vi "Wait Event Callback.vi"(4 "GUI.lvlib:Auto UI.lvlib:Auto UI.lvclass":refnum<class "Auto UI.lvclass">, 5 "Event data":cluster{"showWait":bool}, 6 "CtlRef":refnum<k7>, 7 "Event common data":cluster{"Source":i32, "Type":u32, "Time":u32}) -> ()   [LabVIEW 2023, in "GUI.lvlib" / "Auto UI.lvlib" / "Auto UI.lvclass"]
uses:
  Auto UI.lvclass
  Auto UI.lvclass/Auto UI.ctl
  <vilib>/Utility/cursorutil.llb/Set Cursor (Icon Pict).vi
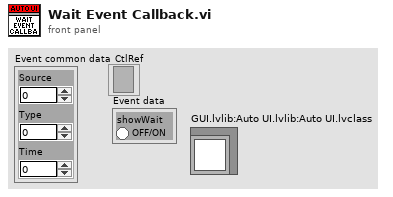
[diagram p1: front panel]
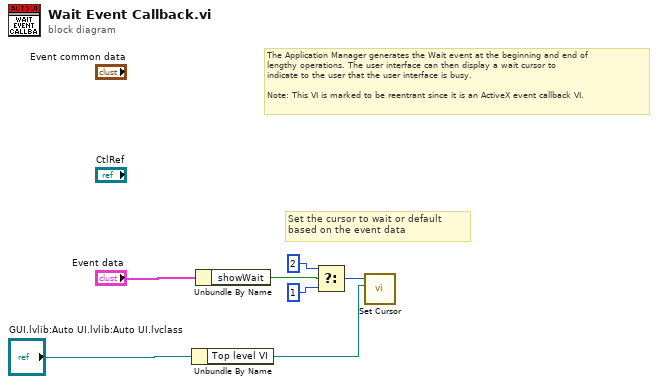
[diagram p0: block diagram]
diagram:
  # "Set the cursor to wait or default based on the event data"
  # "The Application Manager generates the Wait event at the beginning and end of\nlengthy operations. The user interface can then display a wait cursor to\nindicate to the user that the user interface is busy.\n\nNote: This VI is marked to be reentrant since it is an ActiveX event callback VI."
  n1 = Unbundle By Name("GUI.lvlib:Auto UI.lvlib:Auto UI.lvclass") -> ("Top level VI"=w6:refnum<vi>)
  n2 = Unbundle By Name("Event data") -> ("showWait"=w4:bool)
  n3 = Select(t=u16 2 ("icon"), s=w4, f=u16 1 ("icon")) -> (s? t:f=w2:u16)
  n4 = call-poly <vilib>:"Set Cursor.vi"("VI reference (current VI)"=w6, "icon"=w2) -> ()  [unwired: 8 in, 2 out]
